vi "Register gRPC Events.vi"(8 "error in":errorcluster, 11 "Node in":refnum<class "AMS Climate Chamber Template.lvclass">) -> (0 "error out":errorcluster, 2 "Event Registration Refnum":refnum<event-registration>, 3 "Node out":refnum<class "AMS Climate Chamber Template.lvclass">)   [LabVIEW 2023, in "AMS Climate Chamber Template.lvlib" / "AMS Climate Chamber Template.lvclass"]
uses:
  AMS Climate Chamber Template.lvclass
  C:/Program Files/National Instruments/LabVIEW 2024/vi.lib/ADAS Replay HIL/Template Node/Plugin/Template Node/Template Node.lvclass
  Custom gRPC/AMSClimateChamberTemplateService_server/RPC Service/AMSClimateChamberTemplateService/typeDefs/Server gRPC UEs.ctl
  <vilib>/gRPC/LabVIEW gRPC Library/Server API/typeDefs/gRPCId Cluster.ctl
  <vilib>/gRPC/LabVIEW gRPC Library/Shared/grpcId.ctl
  Custom gRPC/AMSClimateChamberTemplateService_server/RPC Service/AMSClimateChamberTemplateService/AMSClimateChamberTemplateService.lvclass
  C:/Program Files/National Instruments/LabVIEW 2024/vi.lib/gRPC/LabVIEW gRPC Servicer/ServiceBase/ServiceBase.lvclass
  Custom gRPC/AMSClimateChamberTemplateService_server/RPC Service/AMSClimateChamberTemplateService/AMSClimateChamberTemplateService.lvclass/AMSClimateChamberTemplateService.ctl
  Custom gRPC/AMSClimateChamberTemplateService_server/RPC Service/AMSClimateChamberTemplateService/Accessor/Read Server RPC Methods.vi
  <vilib>/ADAS Replay HIL/Template Node/Plugin/Template Node/Template Node.lvclass
  <vilib>/gRPC/LabVIEW gRPC Library/grpc-lvsupport-release.lvlib
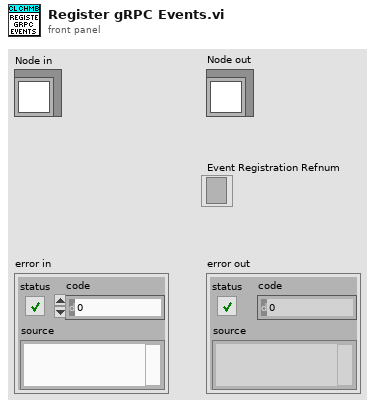
[diagram p1: front panel]
types:
  T1 = typedef "AMSClimateChamberTemplateService_server.lvlib/AMSClimateChamberTemplateService.lvclass/Server gRPC UEs.ctl" = cluster{"BLSClimateChamberTemplateService SetNumber gRPC UE":refnum<user-event>}
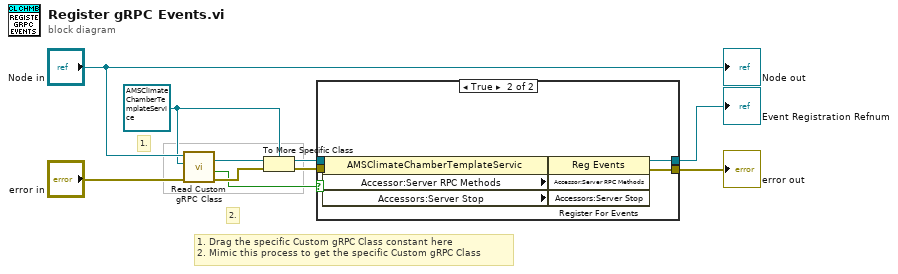
[diagram p0: block diagram]
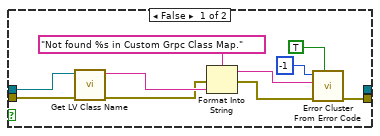
[diagram p2: hidden frame]
diagram:
  w7 = refnum<class "AMSClimateChamberTemplateService.lvclass"> refnum ("NodeCustomService_server.lvlib:NodeCustomService.lvclass")
  # "2."
  # "1."
  # "1. Drag the specific Custom gRPC Class constant here\n2. Mimic this process to get the specific Custom gRPC Class"
  n1 = call <vilib>:"Read Custom gRPC Class.vi"("error in"="error in", "Target Custom gRPC Class"=w7, "Node in"="Node in") -> ("error out"=w5:errorcluster, "Found?"=w1:bool, "Custom gRPC Class out"=w6:refnum<class "ServiceBase.lvclass">)  [unwired: 6 in]
  n2 = To More Specific Class(target class=w7, reference=w6, error in=w5) -> (specific class reference=w3:refnum<class "AMSClimateChamberTemplateService.lvclass">, error out=w2:errorcluster)
  n3 = case shown="True" w1 {
    tunnel: [_ w27] -> w9
    tunnel: [w20 w26] -> w8
    tunnel: w3 -> [w17 w22]
    tunnel: w2 -> [w16 w21]
    frame False {
      n4 = call <vilib>:"Get LV Class Name.vi"("error in (no error)"=w16, "object"=w17) -> ("error out"=w14:errorcluster, "class name"=w15:string)  [unwired: 8 in]
      n5 = Format Into String(format string="Not found %s in Custom Grpc Class Map.", error in=w14, w15) -> (resulting string=w12:string, error out=w13:errorcluster)  [unwired: 1 in]
      n6 = call <vilib>:"Error Cluster From Error Code.vi"("show call chain? (False)"=TRUE, "error in (no error)"=w13, "error message (\"\")"=w12, "error code (0)"=-1) -> ("error out"=w20:errorcluster)  [unwired: 5 in]
    }
    frame True {
      n7 = property class="AMSClimateChamberTemplateServic"(reference=w22, error in=w21) -> (error out=w23:errorcluster, "Accessor:Server RPC Methods"=w25:T1, "Accessors:Server Stop"=w24:refnum<user-event>)  [unwired: 1 out]
      n8 = register-events(error in=w23, w25, w24) -> (reference out=w27:refnum<event-registration>, error out=w26:errorcluster)  [unwired: 1 in]
    }
  }
  "Event Registration Refnum" <- w9
  "error out" <- w8
  "Node out" <- "Node in"
